vi "conversion tester.vi"() -> ()   [LabVIEW 2014]
uses:
  Sensors/BMP180/BMP180 Config Options.ctl
panel:
  out "Temperature (F)":i32 format="%.0f °F"
  out "B6":i32
  out "B7":u32
  out "B4":u32
  out "B3":i32
  out "B5":i32
  out "X3":i32
  out "X2":i32
  out "X1":i32
  out "Pressure":i32 format="%.0f Pa"
  out "Temperature (C)":i32 format="%.0f °C"
  in  "BMP180 Config":T1={"Mode"=enum."Ultra Low Power", "Cal Coefs"={"AC1"={"Addr:"=170, "Val:"=0}, "AC2"={"Addr:"=172, "Val:"=0}, "AC3"={"Addr:"=174, "Val:"=0}, "AC4"={"Addr:"=176, "Val:"=0}, "AC5"={"Addr:"=178, "Val:"=0}, "AC6"={"Addr:"=180, "Val:"=0}, "B1"={"Addr:"=182, "Val:"=0}, "B2"={"Addr:"=184, "Val:"=0}, "MB"={"Addr:"=186, "Val:"=0}, "MC"={"Addr:"=188, "Val:"=0}, "MD"={"Addr:"=190, "Val:"=0}}} {"Cal Coefs"."MD"."Val:" format="%04x"; "Cal Coefs"."MD"."Addr:" format="%02x"; "Cal Coefs"."MC"."Val:" format="%04x"; "Cal Coefs"."MC"."Addr:" format="%02x"; "Cal Coefs"."MB"."Val:" format="%04x"; "Cal Coefs"."MB"."Addr:" format="%02x"; "Cal Coefs"."B2"."Val:" format="%04x"; "Cal Coefs"."B2"."Addr:" format="%02x"; "Cal Coefs"."B1"."Val:" format="%04x"; "Cal Coefs"."B1"."Addr:" format="%02x"; "Cal Coefs"."AC6"."Val:" format="%04x"; "Cal Coefs"."AC6"."Addr:" format="%02x"; "Cal Coefs"."AC5"."Val:" format="%04x"; "Cal Coefs"."AC5"."Addr:" format="%02x"; "Cal Coefs"."AC4"."Val:" format="%04x"; "Cal Coefs"."AC4"."Addr:" format="%02x"; "Cal Coefs"."AC3"."Val:" format="%04x"; "Cal Coefs"."AC3"."Addr:" format="%02x"; "Cal Coefs"."AC2"."Val:" format="%04x"; "Cal Coefs"."AC2"."Addr:" format="%02x"; "Cal Coefs"."AC1"."Val:" format="%04x"; "Cal Coefs"."AC1"."Addr:" format="%02x"}
  # "These values are solely for checking work"
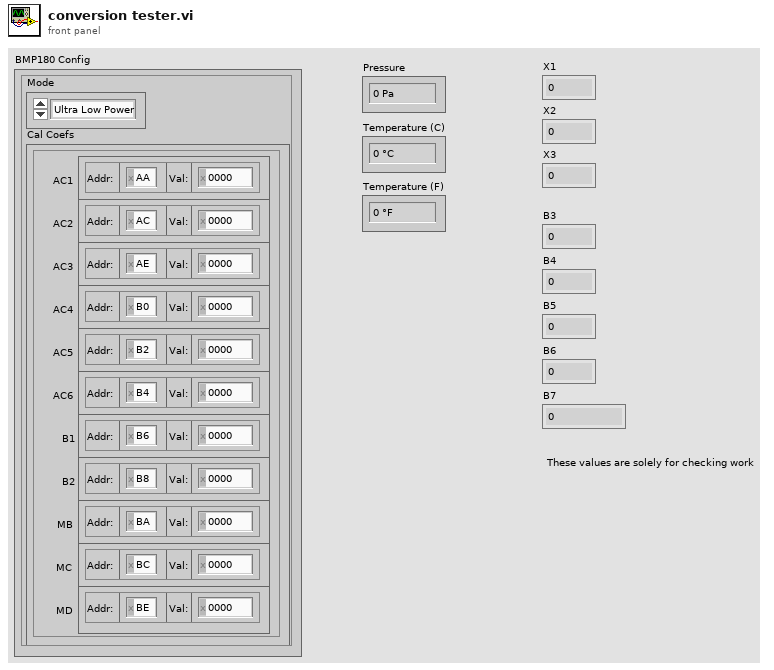
[diagram p1: front panel]
types:
  T1 = typedef "BMP180 Config Options.ctl" = cluster{"Mode":enum8{"Ultra Low Power", "Standard", "High Resolution", "Ultra High Resolution"}, "Cal Coefs":cluster{"AC1":cluster{"Addr:":u8, "Val:":u16}, "AC2":cluster{"Addr:":u8, "Val:":u16}, "AC3":cluster{"Addr:":u8, "Val:":u16}, "AC4":cluster{"Addr:":u8, "Val:":u16}, "AC5":cluster{"Addr:":u8, "Val:":u16}, "AC6":cluster{"Addr:":u8, "Val:":u16}, "B1":cluster{"Addr:":u8, "Val:":u16}, "B2":cluster{"Addr:":u8, "Val:":u16}, "MB":cluster{"Addr:":u8, "Val:":u16}, "MC":cluster{"Addr:":u8, "Val:":u16}, "MD":cluster{"Addr:":u8, "Val:":u16}}}
  T2 = enum8{"Ultra Low Power", "Standard", "High Resolution", "Ultra High Resolution"}
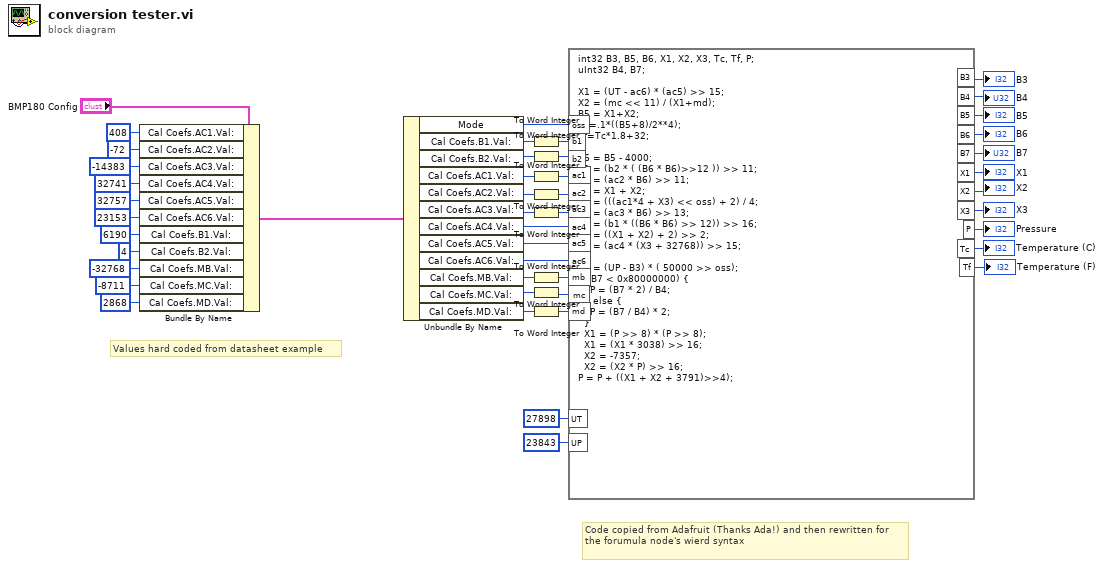
[diagram p0: block diagram]
diagram:
  # "Code copied from Adafruit (Thanks Ada!) and then rewritten for the forumula node's wierd syntax"
  # "Values hard coded from datasheet example"
  n1 = Bundle By Name(cluster="BMP180 Config", "Cal Coefs.AC1.Val:"=i16 408, "Cal Coefs.AC2.Val:"=i16 -72 ("Cal Coefs.AC1.Val:"), "Cal Coefs.AC3.Val:"=i16 -14383 ("Cal Coefs.AC1.Val:"), "Cal Coefs.AC4.Val:"=u16 32741 ("Cal Coefs.AC1.Val:"), "Cal Coefs.AC5.Val:"=u16 32757 ("Cal Coefs.AC1.Val:"), "Cal Coefs.AC6.Val:"=u16 23153 ("Cal Coefs.AC1.Val:"), "Cal Coefs.B1.Val:"=i16 6190 ("Cal Coefs.AC1.Val:"), "Cal Coefs.B2.Val:"=i16 4 ("Cal Coefs.AC1.Val:"), "Cal Coefs.MB.Val:"=i16 -32768 ("Cal Coefs.AC1.Val:"), "Cal Coefs.MC.Val:"=i16 -8711 ("Cal Coefs.AC1.Val:"), "Cal Coefs.MD.Val:"=i16 2868 ("Cal Coefs.AC1.Val:")) -> (w33:T1)
  n2 = Unbundle By Name(w33) -> ("Mode"=w18:T2, "Cal Coefs.B1.Val:"=w19:u16, "Cal Coefs.B2.Val:"=w16:u16, "Cal Coefs.AC1.Val:"=w15:u16, "Cal Coefs.AC2.Val:"=w14:u16, "Cal Coefs.AC3.Val:"=w13:u16, "Cal Coefs.AC4.Val:"=w12:u16, "Cal Coefs.AC5.Val:"=w11:u16, "Cal Coefs.AC6.Val:"=w10:u16, "Cal Coefs.MB.Val:"=w21:u16, "Cal Coefs.MC.Val:"=w7:u16, "Cal Coefs.MD.Val:"=w20:u16)
  n3 = To Word Integer(number=w19) -> (16bit integer=w17:i16)
  n4 = To Word Integer(number=w16) -> (16bit integer=w25:i16)
  n5 = To Word Integer(number=w15) -> (16bit integer=w24:i16)
  n6 = To Word Integer(number=w14) -> (16bit integer=w23:i16)
  n7 = To Word Integer(number=w13) -> (16bit integer=w22:i16)
  n8 = To Word Integer(number=w21) -> (16bit integer=w9:i16)
  n9 = To Word Integer(number=w7) -> (16bit integer=w8:i16)
  n10 = To Word Integer(number=w20) -> (16bit integer=w6:i16)
  n11 = formula code="int32 B3, B5, B6, X1, X2, X3, Tc, Tf, P;\nuInt32 B4, B7;\n\nX1 = (UT - ac6) * (ac5) >> 15;\nX2 = (mc << 11) / (X1+md);\nB5 = X1+X2;\nTc=.1*((B5+8)/2**4);\nTf=Tc*1.8+32;\n\nB6 = B5 - 4000;\nX1 = (b2 * ( (B6 * B6)>>12 )) >> 11;\nX2 = (ac2 * B6) >> 11;\nX3 = X1 + X2;\nB3 = (((ac1*4 + X3) << oss) + 2) / 4;\nX1 = (ac3 * B6) >> 13;\nX2 = (b1 * ((B6 * B6) >> 12)) >> 16;\nX3 = ((X1 + X2) + 2) >> 2;\nB4 = (ac4 * (X3 + 32768)) >> 15;\n  \nB7 = (UP - B3) * ( 50000 >> oss);\nif (B7 < 0x80000000) {\n    P = (B7 * 2) / B4;\n  } else {\n    P = (B7 / B4) * 2;\n  }\n  X1 = (P >> 8) * (P >> 8);\n  X1 = (X1 * 3038) >> 16;\n  X2 = -7357; \n  X2 = (X2 * P) >> 16;\nP = P + ((X1 + X2 + 3791)>>4);"("UT"=27898 ("input variable"), "ac1"=w24, "ac2"=w23, "ac3"=w22, "ac4"=w12, "b2"=w25, "b1"=w17, "oss"=w18, "UP"=23843 ("input variable"), "ac5"=w11, "ac6"=w10, "mb"=w9, "mc"=w8, "md"=w6) -> ("P"=→"Pressure":i32, "X1"=→"X1":i32, "X2"=→"X2":i32, "B5"=→"B5":i32, "B3"=→"B3":i32, "B4"=→"B4":u32, "B6"=→"B6":i32, "X3"=→"X3":i32, "Tc"=→"Temperature (C)":i32, "B7"=→"B7":u32, "Tf"=→"Temperature (F)":i32)
